vi "19572 Series START.vi"(8 "error in (no error)":errorcluster, 11 "VISA resource in":refnum<visa-resource-name>) -> (0 "error out":errorcluster, 3 "VISA resource out":refnum<visa-resource-name>)   [LabVIEW 2015]
panel:
  out "output command":string
  # "START"
  # "This is valid for both:\n19572 & 19052"
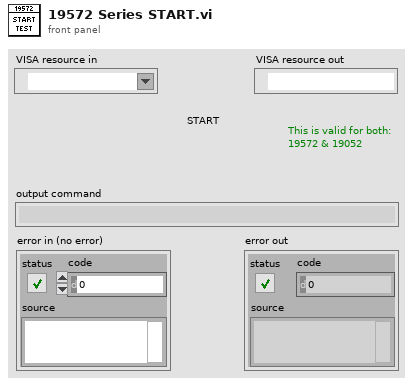
[diagram p1: front panel]
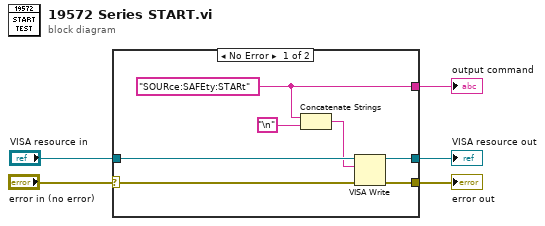
[diagram p0: block diagram]
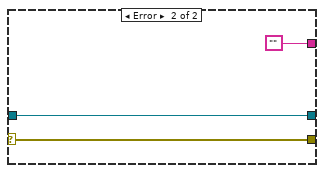
[diagram p2: hidden frame]
diagram:
  n1 = case shown="No Error" "error in (no error)" {
    selector: "error in (no error)" -> [w6 w14]
    tunnel: [w12 w14] -> w5
    tunnel: "VISA resource in" -> [w11 w15]
    tunnel: [w10 w15] -> w3
    tunnel: [w7 ""] -> w2
    frame No Error {
      w7 = "SOURce:SAFEty:STARt"
      n2 = Concatenate Strings(w7, "\n") -> (w8:string)
      n3 = VISA Write(VISA resource name=w11, write buffer=w8, error in (no error)=w6) -> (VISA resource name out=w10:refnum<visa-resource-name>, error out=w12:errorcluster)  [unwired: 1 out]
    }
    frame Error {
    }
  }
  "error out" <- w5
  "VISA resource out" <- w3
  "output command" <- w2
